vi "Columns.vi"() -> (2 "Columns":T1)   [LabVIEW 2020, in "Test.lvlib" / "Game.lvclass"]
uses:
  Game.lvclass
  Columns.ctl
  <vilib>/IlluminatedG/IG Conditum Base/Conditum/Columns/String/String.lvclass
  <vilib>/IlluminatedG/IG Conditum Base/Conditum/Columns/Integer/Integer.lvclass
  <vilib>/IlluminatedG/IG Conditum Base/Conditum/Columns/Boolean/Boolean.lvclass
  <vilib>/IlluminatedG/IG Conditum Base/Conditum/Columns/Double/Double.lvclass
  Game.lvclass/Game.ctl
  <vilib>/IlluminatedG/IG Conditum Base/Conditum/Columns/Type/Definition.ctl
  <vilib>/IlluminatedG/IG Conditum Base/Conditum/Columns/Type/Type.lvclass
  <vilib>/IlluminatedG/IG Conditum Base/Conditum/Attributes.ctl
  <vilib>/IlluminatedG/IG Conditum Base/Conditum/Conditum.lvlib
  <vilib>/IlluminatedG/IG Conditum Base/Conditum/Columns/String/Definition.ctl
  <vilib>/IlluminatedG/IG Conditum Base/Conditum/Columns/String/String Definition.ctl
  <vilib>/IlluminatedG/IG Conditum Base/Conditum/Columns/Integer/Definition.ctl
  <vilib>/IlluminatedG/IG Conditum Base/Conditum/Columns/Integer/Integer Definition.ctl
  <vilib>/IlluminatedG/IG Conditum Base/Conditum/Columns/Boolean/Definition.ctl
  <vilib>/IlluminatedG/IG Conditum Base/Conditum/Columns/Boolean/Boolean Definition.ctl
  <vilib>/IlluminatedG/IG Conditum Base/Conditum/Columns/Double/Definition.ctl
  <vilib>/IlluminatedG/IG Conditum Base/Conditum/Columns/Double/Double Definition.ctl
  C:/Program Files (x86)/National Instruments/LabVIEW 2020/vi.lib/IlluminatedG/IG Conditum Base/Conditum/Columns/Type/Type.lvclass
  C:/Program Files (x86)/National Instruments/LabVIEW 2020/vi.lib/IlluminatedG/IG Conditum Base/Conditum/Columns/String/String.lvclass
  C:/Program Files (x86)/National Instruments/LabVIEW 2020/vi.lib/IlluminatedG/IG Conditum Base/Conditum/Columns/Integer/Integer.lvclass
  C:/Program Files (x86)/National Instruments/LabVIEW 2020/vi.lib/IlluminatedG/IG Conditum Base/Conditum/Columns/Boolean/Boolean.lvclass
  C:/Program Files (x86)/National Instruments/LabVIEW 2020/vi.lib/IlluminatedG/IG Conditum Base/Conditum/Columns/Double/Double.lvclass
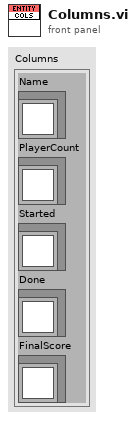
[diagram p1: front panel]
types:
  T1 = typedef "Test.lvlib/Game.lvclass/Columns.ctl" = cluster{"Name":refnum<class "String.lvclass">, "PlayerCount":refnum<class "Integer.lvclass">, "Started":refnum<class "Boolean.lvclass">, "Done":refnum<class "Boolean.lvclass">, "FinalScore":refnum<class "Double.lvclass">}
  T2 = typedef "Conditum.lvlib/Columns.lvlib/Double.lvclass/Double Definition.ctl" = cluster{"Type":T3, "Attributes":T4, "Double":T5}
  T3 = typedef "Conditum.lvlib/Columns.lvlib/Type.lvclass/Definition.ctl" = cluster{"Name":string, "Nullable":bool, "Default NULL":bool}
  T4 = typedef "Conditum.lvlib/Attributes.ctl" = cluster{"Primary Key":bool, "Unique":bool, "Foreign Key":bool, "Auto Increment":bool}
  T5 = typedef "Conditum.lvlib/Columns.lvlib/Double.lvclass/Definition.ctl" = cluster{"Default":dbl}
  T6 = typedef "Conditum.lvlib/Columns.lvlib/Boolean.lvclass/Boolean Definition.ctl" = cluster{"Type":T3, "Attributes":T4, "Boolean":T7}
  T7 = typedef "Conditum.lvlib/Columns.lvlib/Boolean.lvclass/Definition.ctl" = cluster{"Default":bool}
  T8 = typedef "Conditum.lvlib/Columns.lvlib/Integer.lvclass/Integer Definition.ctl" = cluster{"Type":T3, "Attributes":T4, "Integer":T9}
  T9 = typedef "Conditum.lvlib/Columns.lvlib/Integer.lvclass/Definition.ctl" = cluster{"Default":i64}
  T10 = typedef "Conditum.lvlib/Columns.lvlib/String.lvclass/String Definition.ctl" = cluster{"Type":T3, "Attributes":T4, "String":T11}
  T11 = typedef "Conditum.lvlib/Columns.lvlib/String.lvclass/Definition.ctl" = cluster{"Default":string, "Length":i32}
  T12 = cluster{"String out":refnum<class "String.lvclass">, "Integer out":refnum<class "Integer.lvclass">, "Boolean out":refnum<class "Boolean.lvclass">, "Boolean out":refnum<class "Boolean.lvclass">, "Double out":refnum<class "Double.lvclass">}
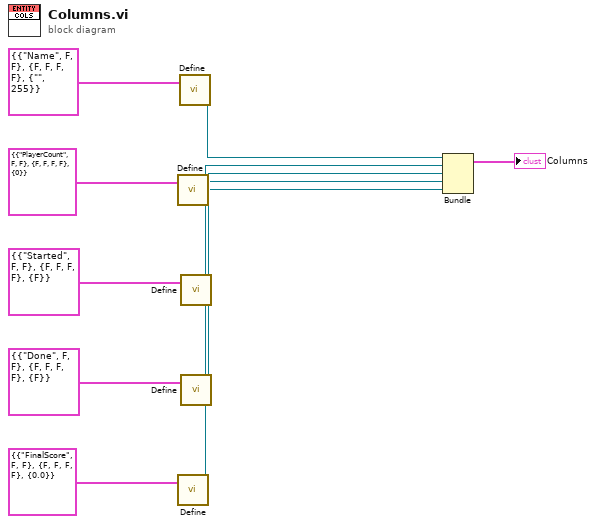
[diagram p0: block diagram]
diagram:
  n1 = call <vilib>:"Define.vi"("Integer Definition"=T8 {"Type"={"Name"="PlayerCount", "Nullable"=FALSE, "Default NULL"=FALSE}, "Attributes"={"Primary Key"=FALSE, "Unique"=FALSE, "Foreign Key"=FALSE, "Auto Increment"=FALSE}, "Integer"={"Default"=0}}) -> ("Integer out"=w7:refnum<class "Integer.lvclass">)  [unwired: 10 in]
  n2 = call <vilib>:"Define.vi"("Double Definition"=T2 {"Type"={"Name"="FinalScore", "Nullable"=FALSE, "Default NULL"=FALSE}, "Attributes"={"Primary Key"=FALSE, "Unique"=FALSE, "Foreign Key"=FALSE, "Auto Increment"=FALSE}, "Double"={"Default"=0.0}}) -> ("Double out"=w1:refnum<class "Double.lvclass">)  [unwired: 10 in]
  n3 = call <vilib>:"Define.vi"("Definition"=T10 {"Type"={"Name"="Name", "Nullable"=FALSE, "Default NULL"=FALSE}, "Attributes"={"Primary Key"=FALSE, "Unique"=FALSE, "Foreign Key"=FALSE, "Auto Increment"=FALSE}, "String"={"Default"="", "Length"=255}}) -> ("String out"=w9:refnum<class "String.lvclass">)  [unwired: 10 in]
  n4 = call <vilib>:"Define.vi"("Init Data"=T6 {"Type"={"Name"="Started", "Nullable"=FALSE, "Default NULL"=FALSE}, "Attributes"={"Primary Key"=FALSE, "Unique"=FALSE, "Foreign Key"=FALSE, "Auto Increment"=FALSE}, "Boolean"={"Default"=FALSE}} ("Definition")) -> ("Boolean out"=w5:refnum<class "Boolean.lvclass">)  [unwired: 10 in]
  n5 = call <vilib>:"Define.vi"("Init Data"=T6 {"Type"={"Name"="Done", "Nullable"=FALSE, "Default NULL"=FALSE}, "Attributes"={"Primary Key"=FALSE, "Unique"=FALSE, "Foreign Key"=FALSE, "Auto Increment"=FALSE}, "Boolean"={"Default"=FALSE}} ("Definition")) -> ("Boolean out"=w3:refnum<class "Boolean.lvclass">)  [unwired: 10 in]
  n6 = Bundle("String out"=w9, "Integer out"=w7, "Boolean out"=w5, "Boolean out"=w3, "Double out"=w1) -> (→"Columns":T12)  [unwired: 1 in]
